vi "Write Layer Table.vi"(8 "Error In":errorcluster, 10 "Layer Information Array":T1 {"Deposition Method" items=["Front Electrode", "Electron Transport Layer", "Active Layer", "Hole Transport Layer", "Back Electrode", "Custom Layer"]; "Layer Type" items=["Front Electrode", "Electron Transport Layer", "Active Layer", "Hole Transport Layer", "Back Electrode", "Custom Layer"]}, 11 "Database Full Information In":T2 {"Database Write Information"."Layer Information Array"."Deposition Method" items=["Blade Coating", "Spin Coating", "Thermal Evaporation", "E-Beam Evaporation", "Sputtering", "Drop Casting", "Dip Coating", "Pulsed Laser Deposition", "Chemival Vapour Deposition", "Atomic Layer Deposition", "Spray Coating", "Screen Printing", "Electroplating", "Molecular Beam Epitaxy", "Custom Deposition"]; "Database Write Information"."Layer Information Array"."Layer Type" items=["Front Electrode", "Electron Transport Layer", "Active Layer", "Hole Transport Layer", "Back Electrode", "Custom Layer"]}) -> (0 "Error Out":errorcluster, 3 "Database Full Information Out":T2 {"Database Write Information"."Layer Information Array"."Deposition Method" items=["Blade Coating", "Spin Coating", "Thermal Evaporation", "E-Beam Evaporation", "Sputtering", "Drop Casting", "Dip Coating", "Pulsed Laser Deposition", "Chemival Vapour Deposition", "Atomic Layer Deposition", "Spray Coating", "Screen Printing", "Electroplating", "Molecular Beam Epitaxy", "Custom Deposition"]; "Database Write Information"."Layer Information Array"."Layer Type" items=["Front Electrode", "Electron Transport Layer", "Active Layer", "Hole Transport Layer", "Back Electrode", "Custom Layer"]})   [LabVIEW 2020]
uses:
  Data Clusters/Database Information.ctl
  Data Clusters/Layer Information Cluster.ctl
  <vilib>/addons/database/Connection.llb/Conn ObjectReference.ctl
  <vilib>/addons/database/NI_Database_API.lvlib
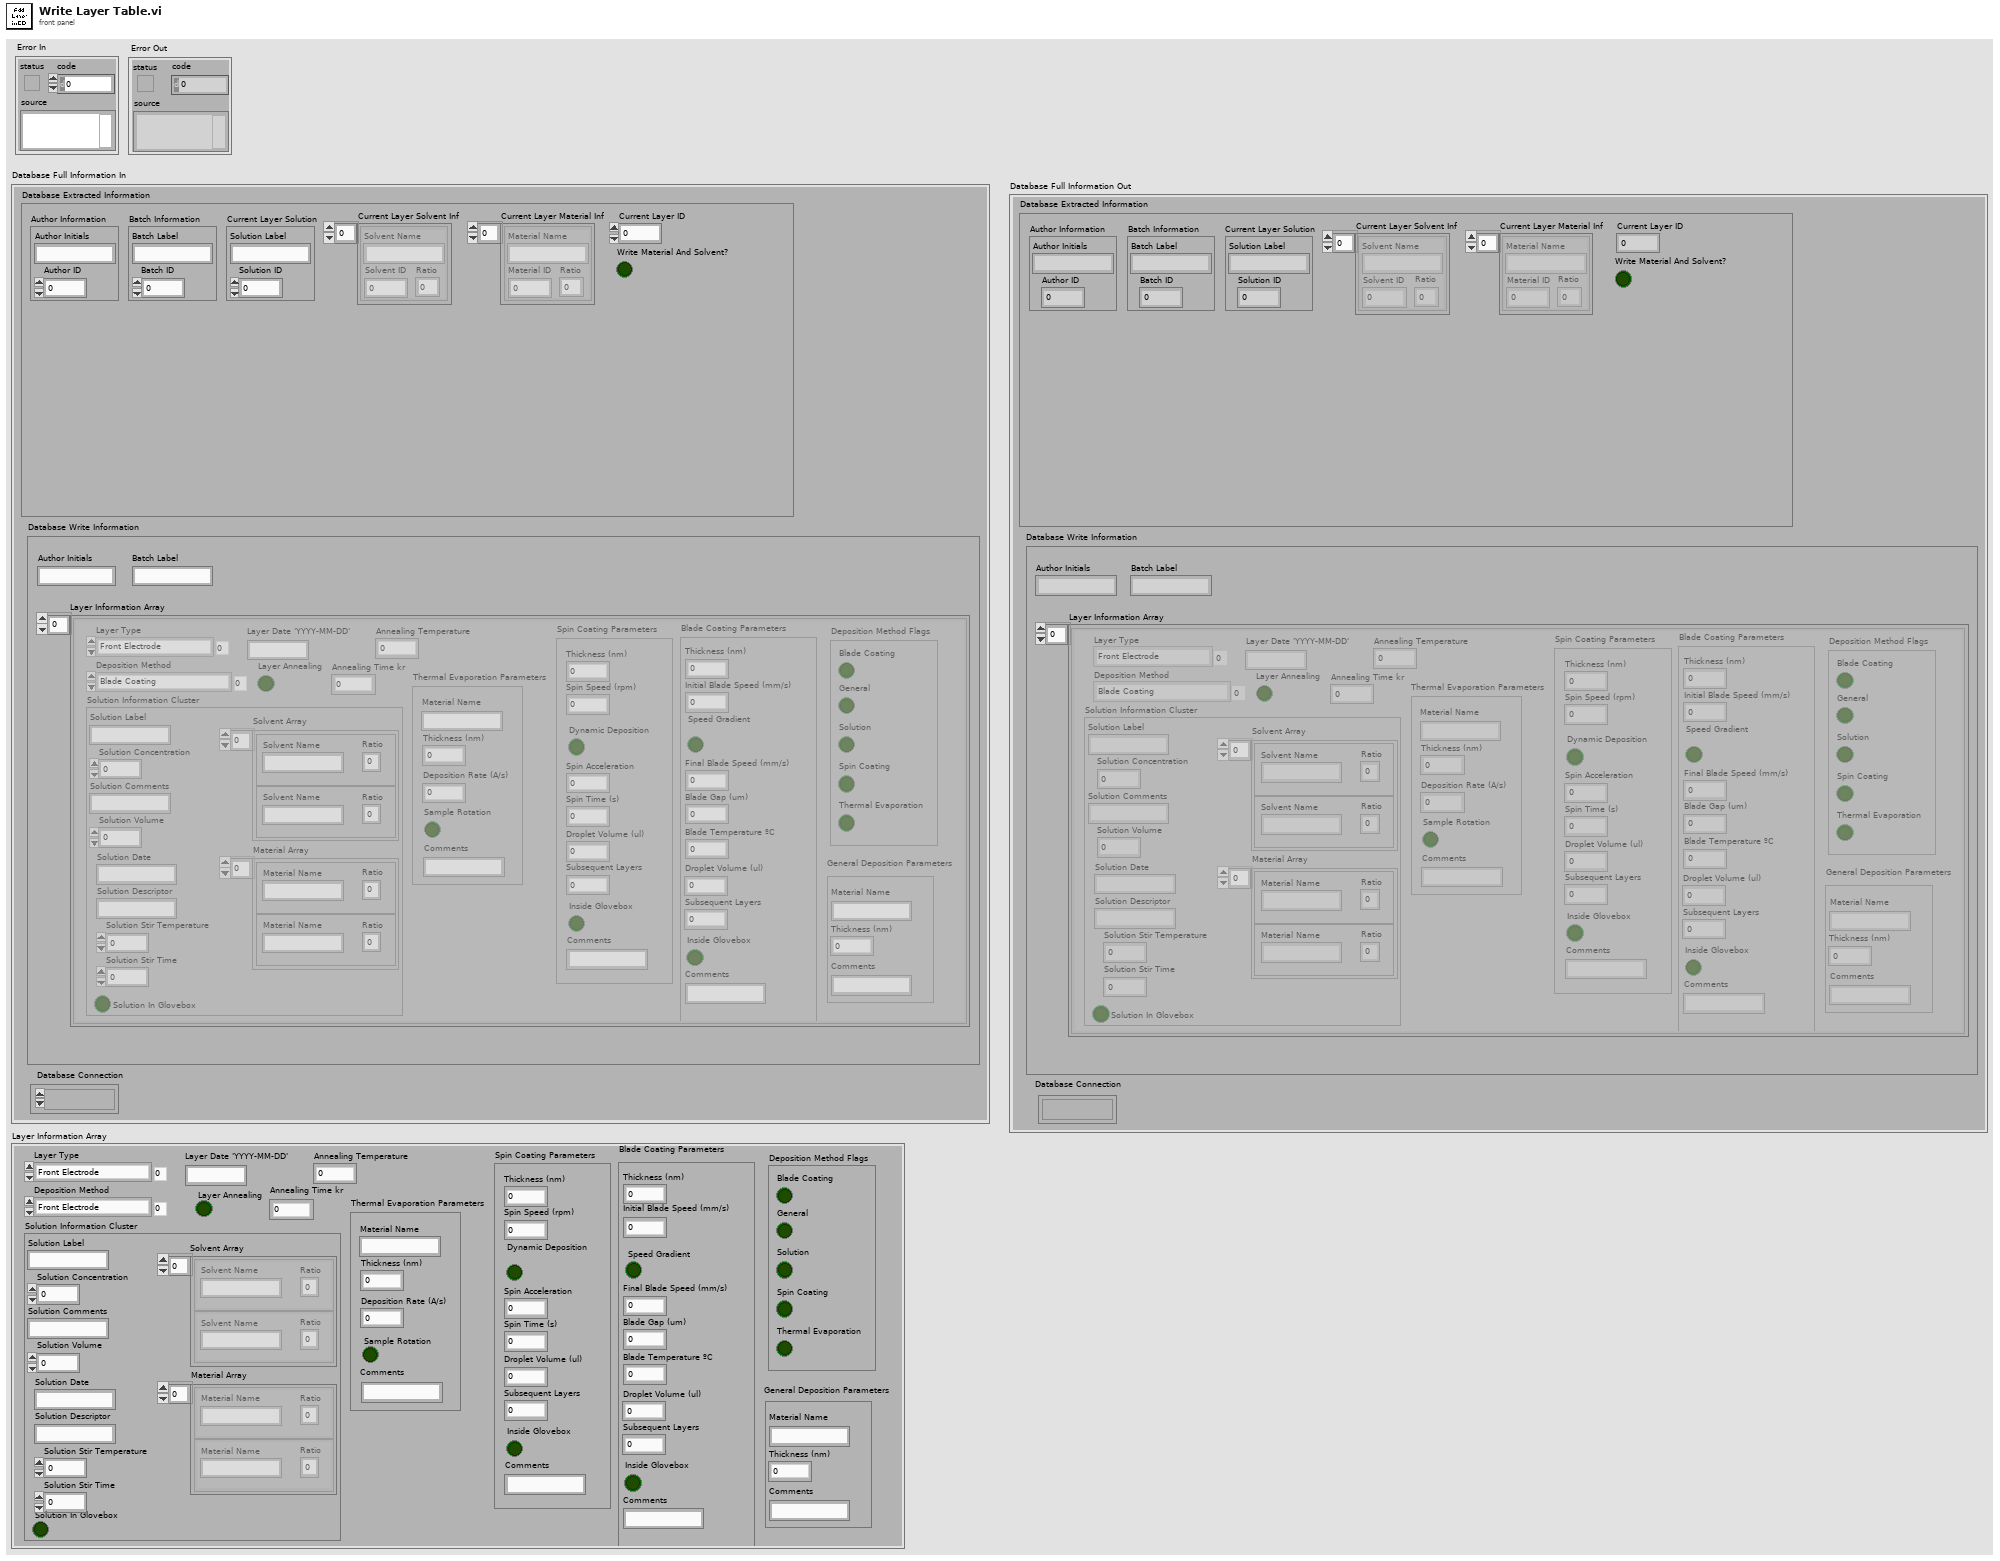
[diagram p1: front panel]
types:
  T1 = typedef "Layer Information Cluster.ctl" = cluster{"Solution Information Cluster":cluster{"Solution Label":string, "Solution Concentration":dbl, "Solution Comments ":string, "Solution Volume ":dbl, "Solution Date ":string, "Solution Descriptor ":string, "Solution Stir Temperature ":dbl, "Solution Stir Time ":dbl, "Solution In Glovebox":bool, "Solvent Array":cluster{"Solvent Name":string, "Ratio":dbl}[], "Material Array":cluster{"Material Name":string, "Ratio":dbl}[]}, "Layer Type":u16, "Deposition Method":u16, "Layer Annealing":bool, "General Deposition Parameters":cluster{"Thickness (nm)":dbl, "Comments":string, "Material Name":string}, "Blade Coating Parameters":cluster{"Thickness (nm)":dbl, "Initial Blade Speed (mm/s)":dbl, "Speed Gradient":bool, "Final Blade Speed (mm/s)":dbl, "Blade Gap (um)":dbl, "Droplet Volume (ul)":dbl, "Subsequent Layers":dbl, "Inside Glovebox":bool, "Comments":string, "Blade Temperature ºC":dbl}, "Spin Coating Parameters":cluster{"Thickness (nm)":dbl, "Spin Speed (rpm)":dbl, "Dynamic Deposition":bool, "Spin Acceleration":dbl, "Spin Time (s)":dbl, "Droplet Volume (ul)":dbl, "Subsequent Layers":dbl, "Inside Glovebox":bool, "Comments":string}, "Thermal Evaporation Parameters":cluster{"Deposition Rate (A/s)":dbl, "Thickness (nm)":dbl, "Comments":string, "Material Name":string, "Sample Rotation":bool}, "Layer Date 'YYYY-MM-DD'":string, "Annealing Time kr":dbl, "Annealing Temperature":dbl, "Deposition Method Flags":cluster{"Blade Coating":bool, "General ":bool, "Solution":bool, "Spin Coating":bool, "Thermal Evaporation":bool}}
  T2 = typedef "Database Information.ctl" = cluster{"Database Extracted Information":cluster{"Author Information":cluster{"Author Initials":string, "Author ID":i32}, "Batch Information":cluster{"Batch Label":string, "Batch ID":i32}, "Current Layer Solution":cluster{"Solution Label":string, "Solution ID":i32}, "Current Layer ID":i32, "Current Layer Solvent Inf":cluster{"Solvent Name":string, "Solvent ID":i32, "Ratio":dbl}[], "Current Layer Material Inf":cluster{"Material Name":string, "Material ID":i32, "Ratio":dbl}[], "Write Material And Solvent?":bool}, "Database Write Information":cluster{"Author Initials":string, "Batch Label":string, "Layer Information Array":T1[]}, "Database Connection":T3}
  T3 = typedef "NI_Database_API.lvlib/Conn ObjectReference.ctl" = refnum<k1>
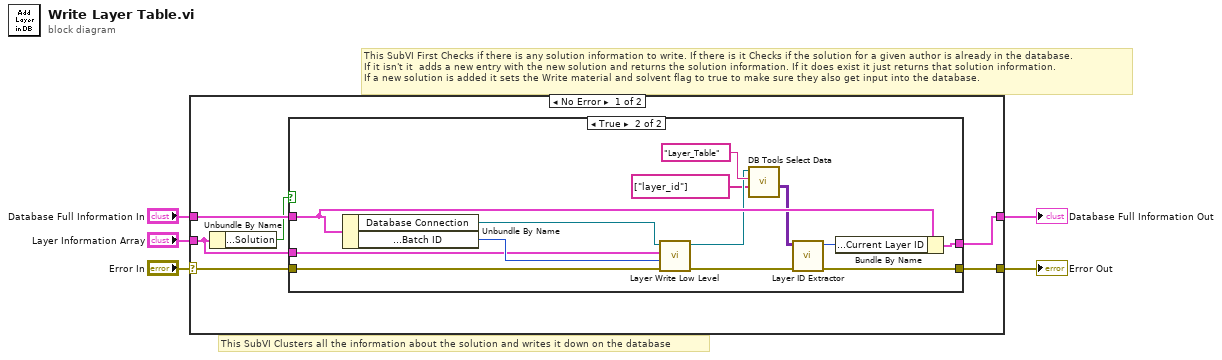
[diagram p0: block diagram]
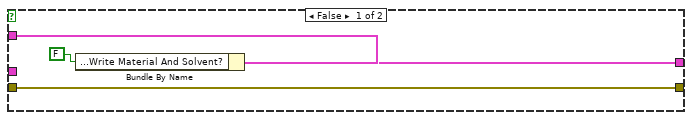
[diagram p2: hidden frame]
diagram:
  # "This SubVI Clusters all the information about the solution and writes it down on the database"
  # "This SubVI First Checks if there is any solution information to write. If there is it Checks if the solution for a given author is already in the database. \nIf it isn't it  adds a new entry with the new solution and returns the solution information. If it does exist it just returns that solution information.\nIf a new solution is added it sets the Write material and solvent flag to true to make sure they also get input into the database."
  n1 = case shown="No Error" "Error In" {
    selector: "Error In" -> [w11 w30]
    tunnel: [w10 w30] -> w4
    tunnel: "Database Full Information In" -> [w9 w29]
    tunnel: [w8 w29] -> w2
    tunnel: "Layer Information Array" -> [w7 _]
    frame No Error {
      n2 = Unbundle By Name(w7) -> ("Deposition Method Flags.Solution"=w6:bool)
      n3 = case shown="True" w6 {
        tunnel: w11 -> [w15 w17]
        tunnel: [w15 w28] -> w10
        tunnel: w9 -> [w14 w27]
        tunnel: [w13 w26] -> w8
        tunnel: w7 -> [_ w24]
        frame False {
          n4 = Bundle By Name(cluster=w14, "Database Extracted Information.Write Material And Solvent?"=FALSE) -> (w13:T2)
        }
        frame True {
          n5 = Unbundle By Name(w27) -> ("Database Connection"=w18:T3, "Database Extracted Information.Batch Information.Batch ID"=w25:i32)
          n6 = call "Layer Write Low Level.vi"("error in (no error)"=w17, "Batch ID"=w25, "Layer Information Cluster"=w24, "Database Connection In"=w18) -> ("error out"=w19:errorcluster, "Database Connection Out"=w22:T3)  [unwired: 6 in]
          n7 = call <vilib>:"DB Tools Select Data.vi"("columns"=string[] ["layer_id"], "table"="Layer_Table", "connection reference"=w22) -> ("data"=w20:variant[][])  [unwired: 3 in, 2 out]
          n8 = call "Layer ID Extractor.vi"("Error In"=w19, "Layer Data"=w20) -> ("Error Out"=w28:errorcluster, "Layer ID"=w16:i32)  [unwired: 8 in]
          n9 = Bundle By Name(cluster=w27, "Database Extracted Information.Current Layer ID"=w16) -> (w26:T2)
        }
      }
    }
    frame Error {
    }
  }
  "Error Out" <- w4
  "Database Full Information Out" <- w2
